vi "PI Controller with Stability Checker.vi"(0 "Loop Rate (s)":dbl format="%#_13g", 1 "Slew Rates":dbl[](array[numeric])=[0.0, 0.0, 0.0], 2 "PI Parameters":T1, 3 "Tolerances":dbl[](array[numeric]), 4 "Feedback":dbl[](array[numeric]), 5 "CtrlIndex":i32, 7 "CommandCluster":T3, 9 "CmdLimits":cluster{"Step":dbl, "Max":dbl, "Min":dbl}, 10 "Loops/step":i32, 11 "Stability In":T2, 12 "Controller?":bool, 13 "FF Scales":dbl[][](array[numeric])=[[0.0, 0.0, 0.0]]) -> (6 "Output":dbl, 8 "PIdata":dbl[](array[numeric]), 14 "Stable?":bool, 15 "Stability Out":T2)   [LabVIEW 2013]
uses:
  TypeDef/Command Cluster.ctl
  TypeDef/PI Parameters.ctl
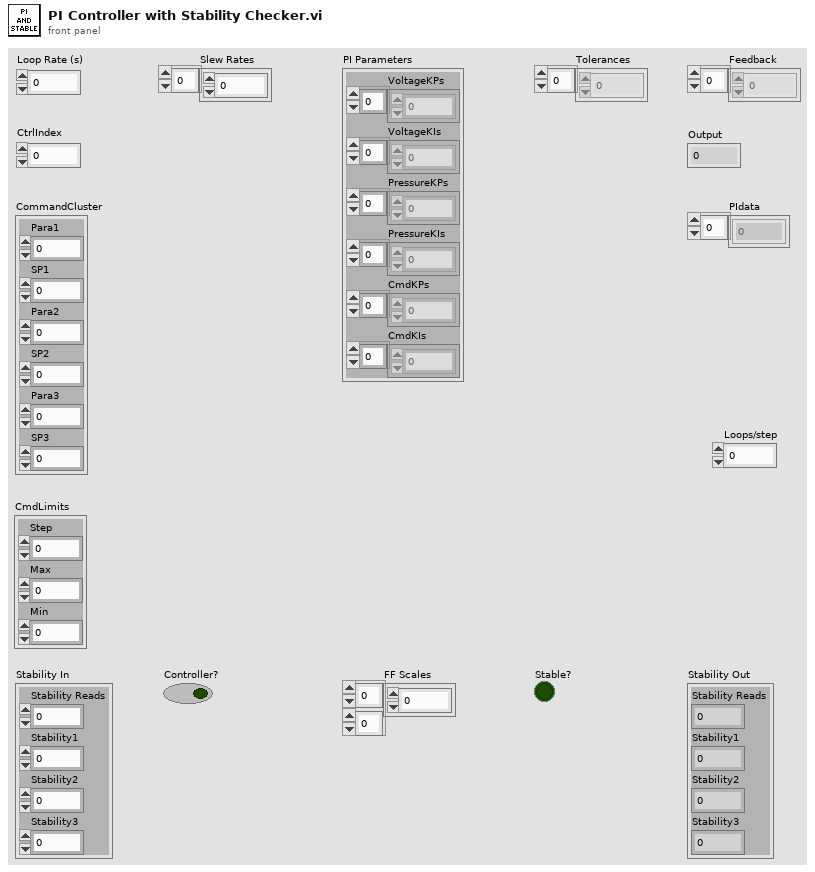
[diagram p1: front panel]
types:
  T1 = typedef "PI Parameters.ctl" = cluster{"VoltageKPs":dbl[], "VoltageKIs":dbl[], "PressureKPs":dbl[], "PressureKIs":dbl[], "CmdKPs":dbl[], "CmdKIs":dbl[]}
  T2 = cluster{"Stability Reads":i32, "Stability1":i32, "Stability2":i32, "Stability3":i32}
  T3 = typedef "Command Cluster.ctl" = cluster{"Para1":i32, "SP1":dbl, "Para2":i32, "SP2":dbl, "Para3":i32, "SP3":dbl}
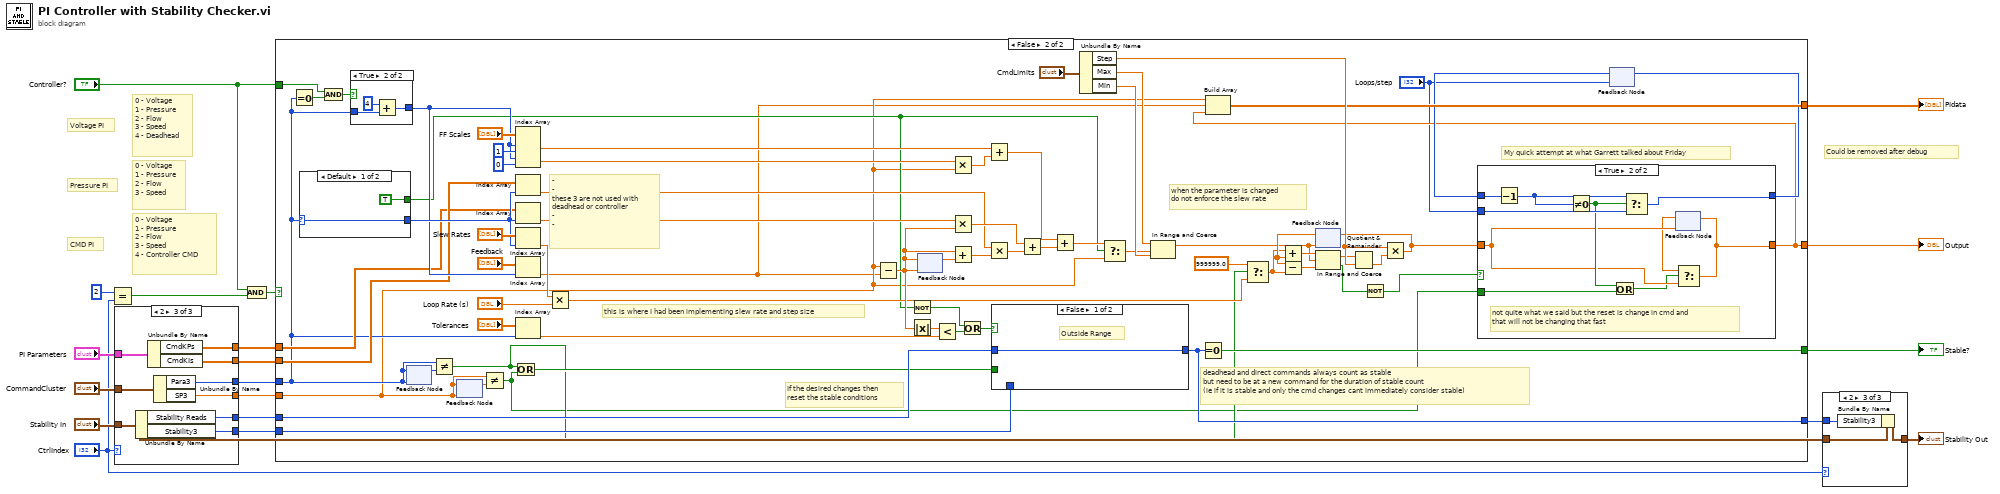
[diagram p0: block diagram]
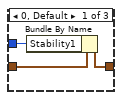
[diagram p2: hidden frame]
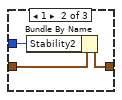
[diagram p3: hidden frame]
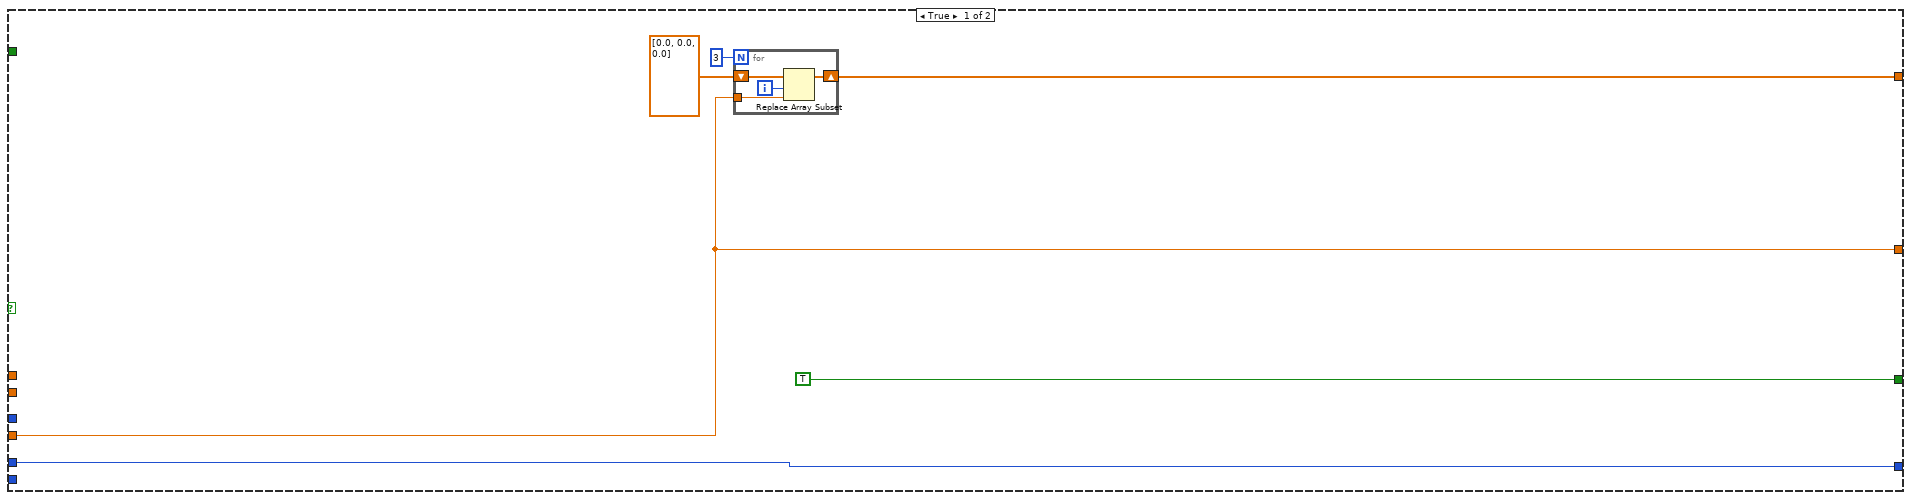
[diagram p4: hidden frame]
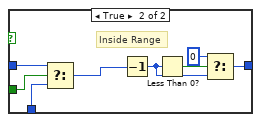
[diagram p7: hidden frame]
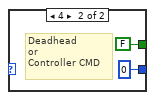
[diagram p8: hidden frame]
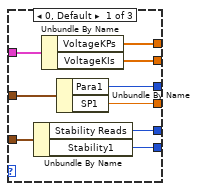
[diagram p9: hidden frame]
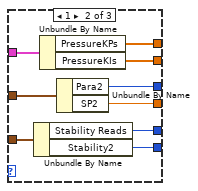
[diagram p10: hidden frame]
diagram:
  # "Could be removed after debug"
  # "CMD PI"
  # "Pressure PI"
  # "Voltage PI"
  # "0 - Voltage\n1 - Pressure\n2 - Flow\n3 - Speed\n4 - Controller CMD"
  # "0 - Voltage\n1 - Pressure\n2 - Flow\n3 - Speed"
  # "0 - Voltage\n1 - Pressure\n2 - Flow\n3 - Speed\n4 - Deadhead"
  n1 = Equal?(x=2, y="CtrlIndex") -> (x = y?=w10:bool)
  n2 = case shown="2" "CtrlIndex" {
    tunnel: "Stability In" -> [w28 w37 w46]
    tunnel: [w26 w35 w44] -> w18
    tunnel: [w27 w36 w45] -> w17
    tunnel: "CommandCluster" -> [w25 w34 w43]
    tunnel: [w24 w33 w42] -> w13
    tunnel: [w23 w32 w41] -> w12
    tunnel: "PI Parameters" -> [w22 w29 w40]
    tunnel: [w21 w31 w39] -> w14
    tunnel: [w20 w30 w38] -> w15
    frame 0, Default {
      n3 = Unbundle By Name(w28) -> ("Stability Reads"=w26:i32, "Stability1"=w27:i32)
      n4 = Unbundle By Name(w22) -> ("VoltageKPs"=w21:dbl[], "VoltageKIs"=w20:dbl[])
      n5 = Unbundle By Name(w25) -> ("Para1"=w24:i32, "SP1"=w23:dbl)
    }
    frame 1 {
      n6 = Unbundle By Name(w37) -> ("Stability Reads"=w35:i32, "Stability2"=w36:i32)
      n7 = Unbundle By Name(w29) -> ("PressureKPs"=w31:dbl[], "PressureKIs"=w30:dbl[])
      n8 = Unbundle By Name(w34) -> ("Para2"=w33:i32, "SP2"=w32:dbl)
    }
    frame 2 {
      n9 = Unbundle By Name(w46) -> ("Stability Reads"=w44:i32, "Stability3"=w45:i32)
      n10 = Unbundle By Name(w40) -> ("CmdKPs"=w39:dbl[], "CmdKIs"=w38:dbl[])
      n11 = Unbundle By Name(w43) -> ("Para3"=w42:i32, "SP3"=w41:dbl)
    }
  }
  n12 = And(x="Controller?", y=w10) -> (x .and. y?=w8:bool)
  n13 = case shown="False" w8 {
    tunnel: w18 -> [w51 w94]
    tunnel: w17 -> [_ w93]
    tunnel: w15 -> [_ w92]
    tunnel: w14 -> [_ w91]
    tunnel: w13 -> [_ w83]
    tunnel: w12 -> [w50 w68]
    tunnel: "Controller?" -> [_ w74]
    tunnel: [TRUE w73] -> w6
    tunnel: [w50 w60] -> w5
    tunnel: [w48 w72] -> w4
    tunnel: [w51 w71] -> w3
    frame True {
      n14 = for {
        N: 3 -> [_]
        shift-right: [w55] -> w48
        shift-left: dbl[] [0.0, 0.0, 0.0] -> [w56]
        tunnel: w50 -> [w53]
        i -> [w54]
        n15 = Replace Array Subset(array=w56, new element=w53, index=w54) -> (w55:dbl[])
      }
    }
    frame False {
      # "My quick attempt at what Garrett talked about Friday"
      # "this is where I had been implementing slew rate and step size"
      # "-\n-\nthese 3 are not used with\ndeadhead or controller\n-\n-"
      # "deadhead and direct commands always count as stable\nbut need to be at a new command for the duration of stable count\n(ie if it is stable and only the cmd changes cant immediately consider stable)"
      # "when the parameter is changed\ndo not enforce the slew rate"
      # "If the desired changes then\nreset the stable conditions"
      n16 = Equal To 0?(x=w83) -> (x = 0?=w99:bool)
      n17 = case shown="Default" w83 {
        selector: w83 -> [w150 _]
        tunnel: [w150 0 ("index")] -> w97
        tunnel: [TRUE FALSE] -> w78
        frame Default {
        }
        frame 4 {
          # "Deadhead\nor\nController CMD"
        }
      }
      n18 = And(x=w74, y=w99) -> (x .and. y?=w98:bool)
      n19 = case shown="True" w98 {
        tunnel: w83 -> [w137 w140]
        tunnel: [w137 w138] -> w95
        frame False {
        }
        frame True {
          n20 = Add(x=4, y=w140) -> (x+y=w138:i32)
        }
      }
      n21 = feedback #1(w83) -> (w85:i32)
      n22 = feedback-in #1(w83) -> ()
      n23 = Not Equal?(x=w83, y=w85) -> (x != y?=w67:bool)
      n24 = feedback #2(w68) -> (w84:dbl)
      n25 = feedback-in #2(w68) -> ()
      n26 = Not Equal?(x=w68, y=w84) -> (x != y?=w61:bool)
      n27 = Or(x=w67, y=w61) -> (x .or. y?=w82:bool)
      n28 = Index Array(array="FF Scales", index (row) #1=w95, index (col) #1=1 ("disabled index (col)"), index (row) #2=w95, index (col) #2=0 ("disabled index (col)")) -> (element #1=w104:dbl, element #2=w112:dbl)
      n29 = Index Array(array=w92, index=w97) -> (element=w119:dbl)
      n30 = Index Array(array=w91, index=w97) -> (element=w121:dbl)
      n31 = Index Array(array="Slew Rates", index=w97) -> (element=w101:dbl)
      n32 = Index Array(array="Feedback", index=w95) -> (element=w65:dbl)
      n33 = Index Array(array="Tolerances", index=w83) -> (element=w122:dbl)
      n34 = Multiply(x=w101, y="Loop Rate (s)") -> (x*y=w81:dbl)
      n35 = Subtract(x=w68, y=w65) -> (x-y=w115:dbl)
      n36 = Not(x=w78) -> (.not. x?=w77:bool)
      n37 = Absolute Value(x=w115) -> (abs(x)=w123:dbl)
      n38 = feedback #3(w115) -> (w116:dbl)
      n39 = feedback-in #3(w115) -> ()
      n40 = Less?(x=w123, y=w122) -> (x < y?=w76:bool)
      n41 = Multiply(x=w112, y=w68) -> (x*y=w105:dbl)
      n42 = Multiply(x=w121, y=w115) -> (x*y=w120:dbl)
      n43 = Add(x=w115, y=w116) -> (x+y=w117:dbl)
      n44 = Or(x=w77, y=w76) -> (x .or. y?=w75:bool)
      n45 = Add(x=w104, y=w105) -> (x+y=w103:dbl)
      n46 = Multiply(x=w119, y=w117) -> (x*y=w118:dbl)
      n47 = case shown="False" w75 {
        tunnel: [w141 w146] -> w71
        tunnel: w94 -> [w141 w144]
        tunnel: w93 -> [_ w143]
        tunnel: w82 -> [_ w145]
        frame False {
          # "Outside Range"
        }
        frame True {
          # "Inside Range"
          n48 = Select(t=w144, s=w145, f=w143) -> (s? t:f=w142:i32)
          n49 = Decrement(x=w142) -> (x-1=w148:i32)
          n50 = Less Than 0?(x=w148) -> (x < 0?=w147:bool)
          n51 = Select(t=0, s=w147, f=w148) -> (s? t:f=w146:i32)
        }
      }
      n52 = Add(x=w120, y=w118) -> (x+y=w111:dbl)
      n53 = Add(x=w103, y=w111) -> (x+y=w100:dbl)
      n54 = Unbundle By Name("CmdLimits") -> ("Step"=w87:dbl, "Max"=w88:dbl, "Min"=w89:dbl)
      n55 = Select(t=w100, s=w78, f=w68) -> (s? t:f=w69:dbl)
      n56 = In Range and Coerce(upper limit=w88, x=w69, lower limit=w89) -> (coerced(x)=w66:dbl)  [unwired: 1 out]
      n57 = Equal To 0?(x=w71) -> (x = 0?=w73:bool)
      n58 = Select(t=999999.0, s=w67, f=w81) -> (s? t:f=w80:dbl)
      n59 = feedback #4(w66) -> (w108:dbl)
      n60 = Add(x=w80, y=w108) -> (x+y=w110:dbl)
      n61 = Subtract(x=w108, y=w80) -> (x-y=w109:dbl)
      n62 = In Range and Coerce(upper limit=w110, x=w66, lower limit=w109) -> (coerced(x)=w70:dbl, In Range?=w59:bool)
      n63 = Quotient & Remainder(x=w70, y=w87) -> (floor(x/y)=w86:dbl)  [unwired: 1 out]
      n64 = Not(x=w59) -> (.not. x?=w58:bool)
      n65 = Multiply(x=w87, y=w86) -> (x*y=w64:dbl)
      n66 = feedback-in #4(w64) -> ()
      n67 = feedback #5("Loops/step") -> (w62:i32)
      n68 = case shown="True" w58 {
        tunnel: w64 -> [w126 w129]
        tunnel: [w126 w132] -> w60
        tunnel: [w125 w135] -> w63
        tunnel: w62 -> [_ w136]
        tunnel: "Loops/step" -> [w125 w133]
        tunnel: w61 -> [_ w131]
        frame False {
        }
        frame True {
          # "not quite what we said but the reset is change in cmd and\nthat will not be changing that fast"
          n69 = Decrement(x=w136) -> (x-1=w134:i32)
          n70 = Not Equal To 0?(x=w134) -> (x != 0?=w130:bool)
          n71 = Or(x=w130, y=w131) -> (x .or. y?=w127:bool)
          n72 = Select(t=w134, s=w130, f=w133) -> (s? t:f=w135:i32)
          n73 = feedback #6(w129) -> (w128:dbl)
          n74 = Select(t=w128, s=w127, f=w129) -> (s? t:f=w132:dbl)
          n75 = feedback-in #6(w132) -> ()
        }
      }
      n76 = Build Array(w68, w65, w60) -> (w72:dbl[])
      n77 = feedback-in #5(w63) -> ()
    }
  }
  "Stable?" <- w6
  "Output" <- w5
  "PIdata" <- w4
  n78 = case shown="2" "CtrlIndex" {
    tunnel: "Stability In" -> [w155 w158 w161]
    tunnel: [w154 w157 w160] -> w7
    tunnel: w3 -> [w156 w159 w162]
    frame 0, Default {
      n79 = Bundle By Name(cluster=w155, "Stability1"=w156) -> (w154:T2)
    }
    frame 1 {
      n80 = Bundle By Name(cluster=w158, "Stability2"=w159) -> (w157:T2)
    }
    frame 2 {
      n81 = Bundle By Name(cluster=w161, "Stability3"=w162) -> (w160:T2)
    }
  }
  "Stability Out" <- w7
